vi "Init Async State Vars.vi"(8 "Error in":errorcluster, 10 "Async Parameters":T5) -> (0 "Error out":errorcluster, 3 "Async State Vars":T1)   [LabVIEW 2015, in "Waveform-Processing-Custom-Device Engine.lvlib"]
uses:
  Waveform-Processing-Custom-Device Engine.lvlib
  <vilib>/NI Veristand/Custom Device Waveform API/Single Waveform Read (DBL)/Single Waveform Read (DBL).lvclass
  <vilib>/NI Veristand/Custom Device Waveform API/Single Waveform Write (DBL)/Single Waveform Write (DBL).lvclass
  <vilib>/NI Veristand/Custom Device API/Waveform Data Reference.ctl
  <vilib>/NI VeriStand/Custom Device API/Custom Device API.lvlib
  Types/AsyncStateVariables.ctl
  <vilib>/ni/NIVS Inline Async API/_Data Access Engine/Access Type Classes/Read/Read.lvclass
  <vilib>/ni/NIVS Inline Async API/_Data Access Engine/Data Access Engine/Types/Read.DVR.ctl
  <vilib>/ni/NIVS Inline Async API/_Data Access Engine/Data Access Engine/Data Access Engine.lvclass
  <vilib>/ni/NIVS Inline Async API/_Data Access Engine/Access Type Classes/Write/Write.lvclass
  <vilib>/ni/NIVS Inline Async API/_Data Access Engine/Data Access Engine/Types/Write.DVR.ctl
  Types/Async FIFOs.ctl
  Types/Async Parameters.ctl
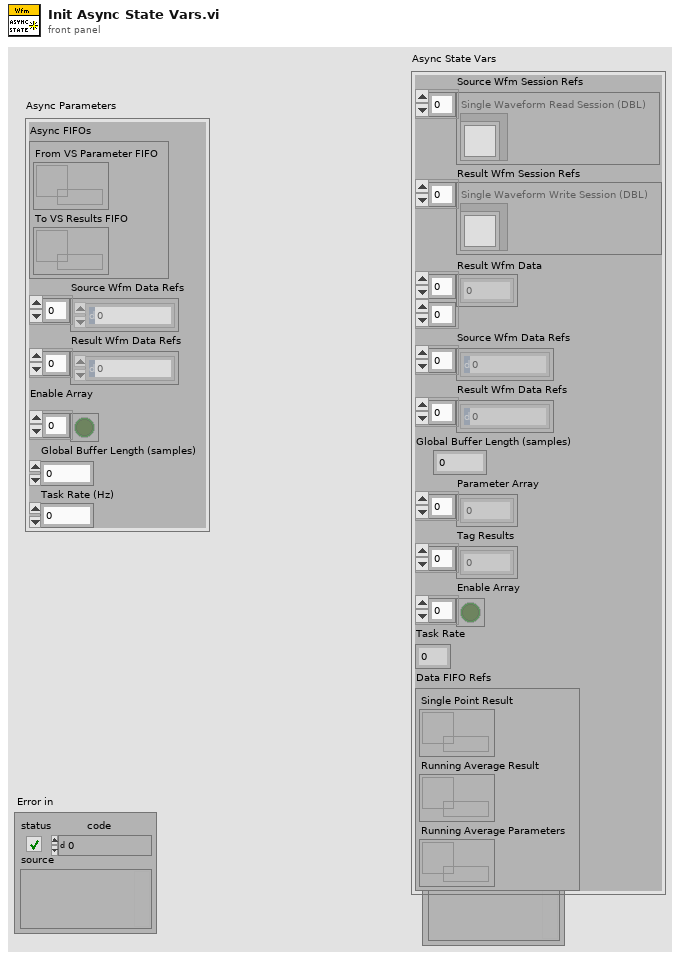
[diagram p1: front panel]
types:
  T1 = typedef "Waveform-Processing-Custom-Device Engine.lvlib/AsyncStateVariables.ctl" = cluster{"Source Wfm Session Refs":refnum<class "Single Waveform Read (DBL).lvclass">[], "Result Wfm Session Refs":refnum<class "Single Waveform Write (DBL).lvclass">[], "Result Wfm Data":dbl[][], "Source Wfm Data Refs":T2[], "Result Wfm Data Refs":T2[], "Global Buffer Length (samples)":dbl, "Parameter Array":dbl[], "Tag Results":dbl[], "Enable Array":bool[], "Task Rate":dbl, "Data FIFO Refs":cluster{"Single Point Result":T3, "Running Average Result":T3, "Running Average Parameters":T4}}
  T2 = typedef "Custom Device API.lvlib/Waveform Data Reference.ctl" = i32
  T3 = typedef "Data Access Engine.lvlib/Data Access Engine.lvclass/Write.DVR.ctl" = refnum<data-value>
  T4 = typedef "Data Access Engine.lvlib/Data Access Engine.lvclass/Read.DVR.ctl" = refnum<data-value>
  T5 = typedef "Waveform-Processing-Custom-Device Engine.lvlib/Async Parameters.ctl" = cluster{"Async FIFOs":T6, "Source Wfm Data Refs":T2[], "Result Wfm Data Refs":T2[], "Enable Array":bool[], "Global Buffer Length (samples)":dbl, "Task Rate (Hz)":dbl}
  T6 = typedef "Waveform-Processing-Custom-Device Engine.lvlib/Async FIFOs.ctl" = cluster{"From VS Parameter FIFO":refnum<k33>, "To VS Results FIFO":refnum<k33>}
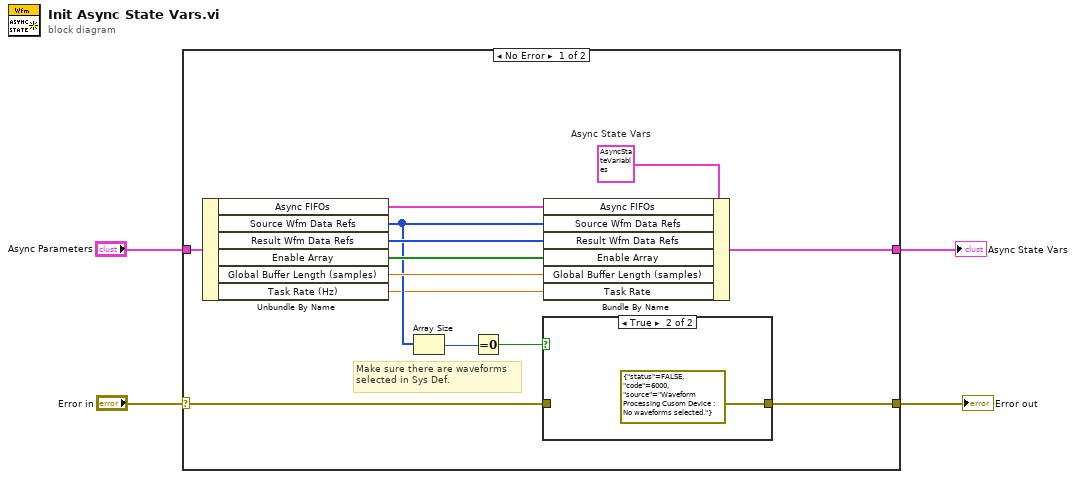
[diagram p0: block diagram]
diagram:
  n1 = case shown="No Error" "Error in" {
    selector: "Error in" -> [w7 w20]
    tunnel: [w6 w20] -> w3
    tunnel: "Async Parameters" -> [w17 _]
    tunnel: [w13 _] -> w1
    frame No Error {
      w16 = T1 {"Source Wfm Session Refs"=[], "Result Wfm Session Refs"=[], "Result Wfm Data"=[], "Source Wfm Data Refs"=[], "Result Wfm Data Refs"=[], "Global Buffer Length (samples)"=0.0, "Parameter Array"=[], "Tag Results"=[], "Enable Array"=[], "Task Rate"=0.0, "Data FIFO Refs"={"Single Point Result"=refnum, "Running Average Result"=refnum, "Running Average Parameters"=refnum}}  # Async State Vars
      # "Make sure there are waveforms\nselected in Sys Def."
      n2 = Unbundle By Name(w17) -> ("Async FIFOs"=w15:T6, "Source Wfm Data Refs"=w10:T2[], "Result Wfm Data Refs"=w14:T2[], "Enable Array"=w12:bool[], "Global Buffer Length (samples)"=w11:dbl, "Task Rate (Hz)"=w5:dbl)
      n3 = Array Size(array=w10) -> (size(s)=w9:i32)
      n4 = Equal To 0?(x=w9) -> (x = 0?=w8:bool)
      n5 = case shown="True" w8 {
        tunnel: w7 -> [w18 _]
        tunnel: [w18 errorcluster {"status"=FALSE, "code"=6000, "source"="Waveform Processing Cusom Device : No waveforms selected."} ("error IO")] -> w6
        frame False {
        }
        frame True {
        }
      }
      n6 = Bundle By Name(cluster=w16, "Async FIFOs"=w15, "Source Wfm Data Refs"=w10, "Result Wfm Data Refs"=w14, "Enable Array"=w12, "Global Buffer Length (samples)"=w11, "Task Rate"=w5) -> (w13:T1)
    }
    frame Error {
    }
  }
  "Error out" <- w3
  "Async State Vars" <- w1
